vi "LoadAndAlignMulti.vi"(8 "error in (no error)":errorcluster, 11 "FileList":string[][](array[string])) -> (0 "error out":errorcluster, 3 "AllDataArray":T1[](array[typedef]) {"FlukeData"."DataAnalysisArray"."TimeStamp" format="%^<%.3X\n%x>T"; "FlukeData"."ModelDataArray"."FREQUENCY" format="%#_6f"; "FlukeData"."ModelDataArray"."TimeStamp" format="%^<%.3X\n%x>T"; "FlukeData"."PMUDataArray"."FREQUENCY" format="%#_6f"; "FlukeData"."PMUDataArray"."TimeStamp" format="%^<%.3X\n%x>T"; "NISTData"."DataAnlysisArray"."Time" format="%.6f"; "NISTData"."DataAnlysisArray"."TimeStamp" format="%^<%.3X\n%x>T"; "NISTData"."DUTDataArray"."TimeStamp" format="%^<%.3X\n%x>T"; "NISTData"."DUTDataArray"."Time" format="%.6f"; "NISTData"."NIDataArray"."TimeStamp" format="%^<%.3X\n%x>T"; "NISTData"."NIDataArray"."Time" format="%.6f"})   [LabVIEW 2014]
uses:
  typedefs/NIData.ctl
  typedefs/NIDataArray.ctl
  typedefs/PhasorRectangular.ctl
  typedefs/PmuRawDataCluster.ctl
  typedefs/CalcPhasorError.ctl
  typedefs/CalcAnalysis.ctl
  typedefs/PlotDataArrays.ctl
  typedefs/DUTData.ctl
  typedefs/NISTData.ctl
  typedefs/Alldata.ctl
  typedefs/NICalcAnalysis.ctl
  Fluke(lib)/Fluke(lib).lvlib
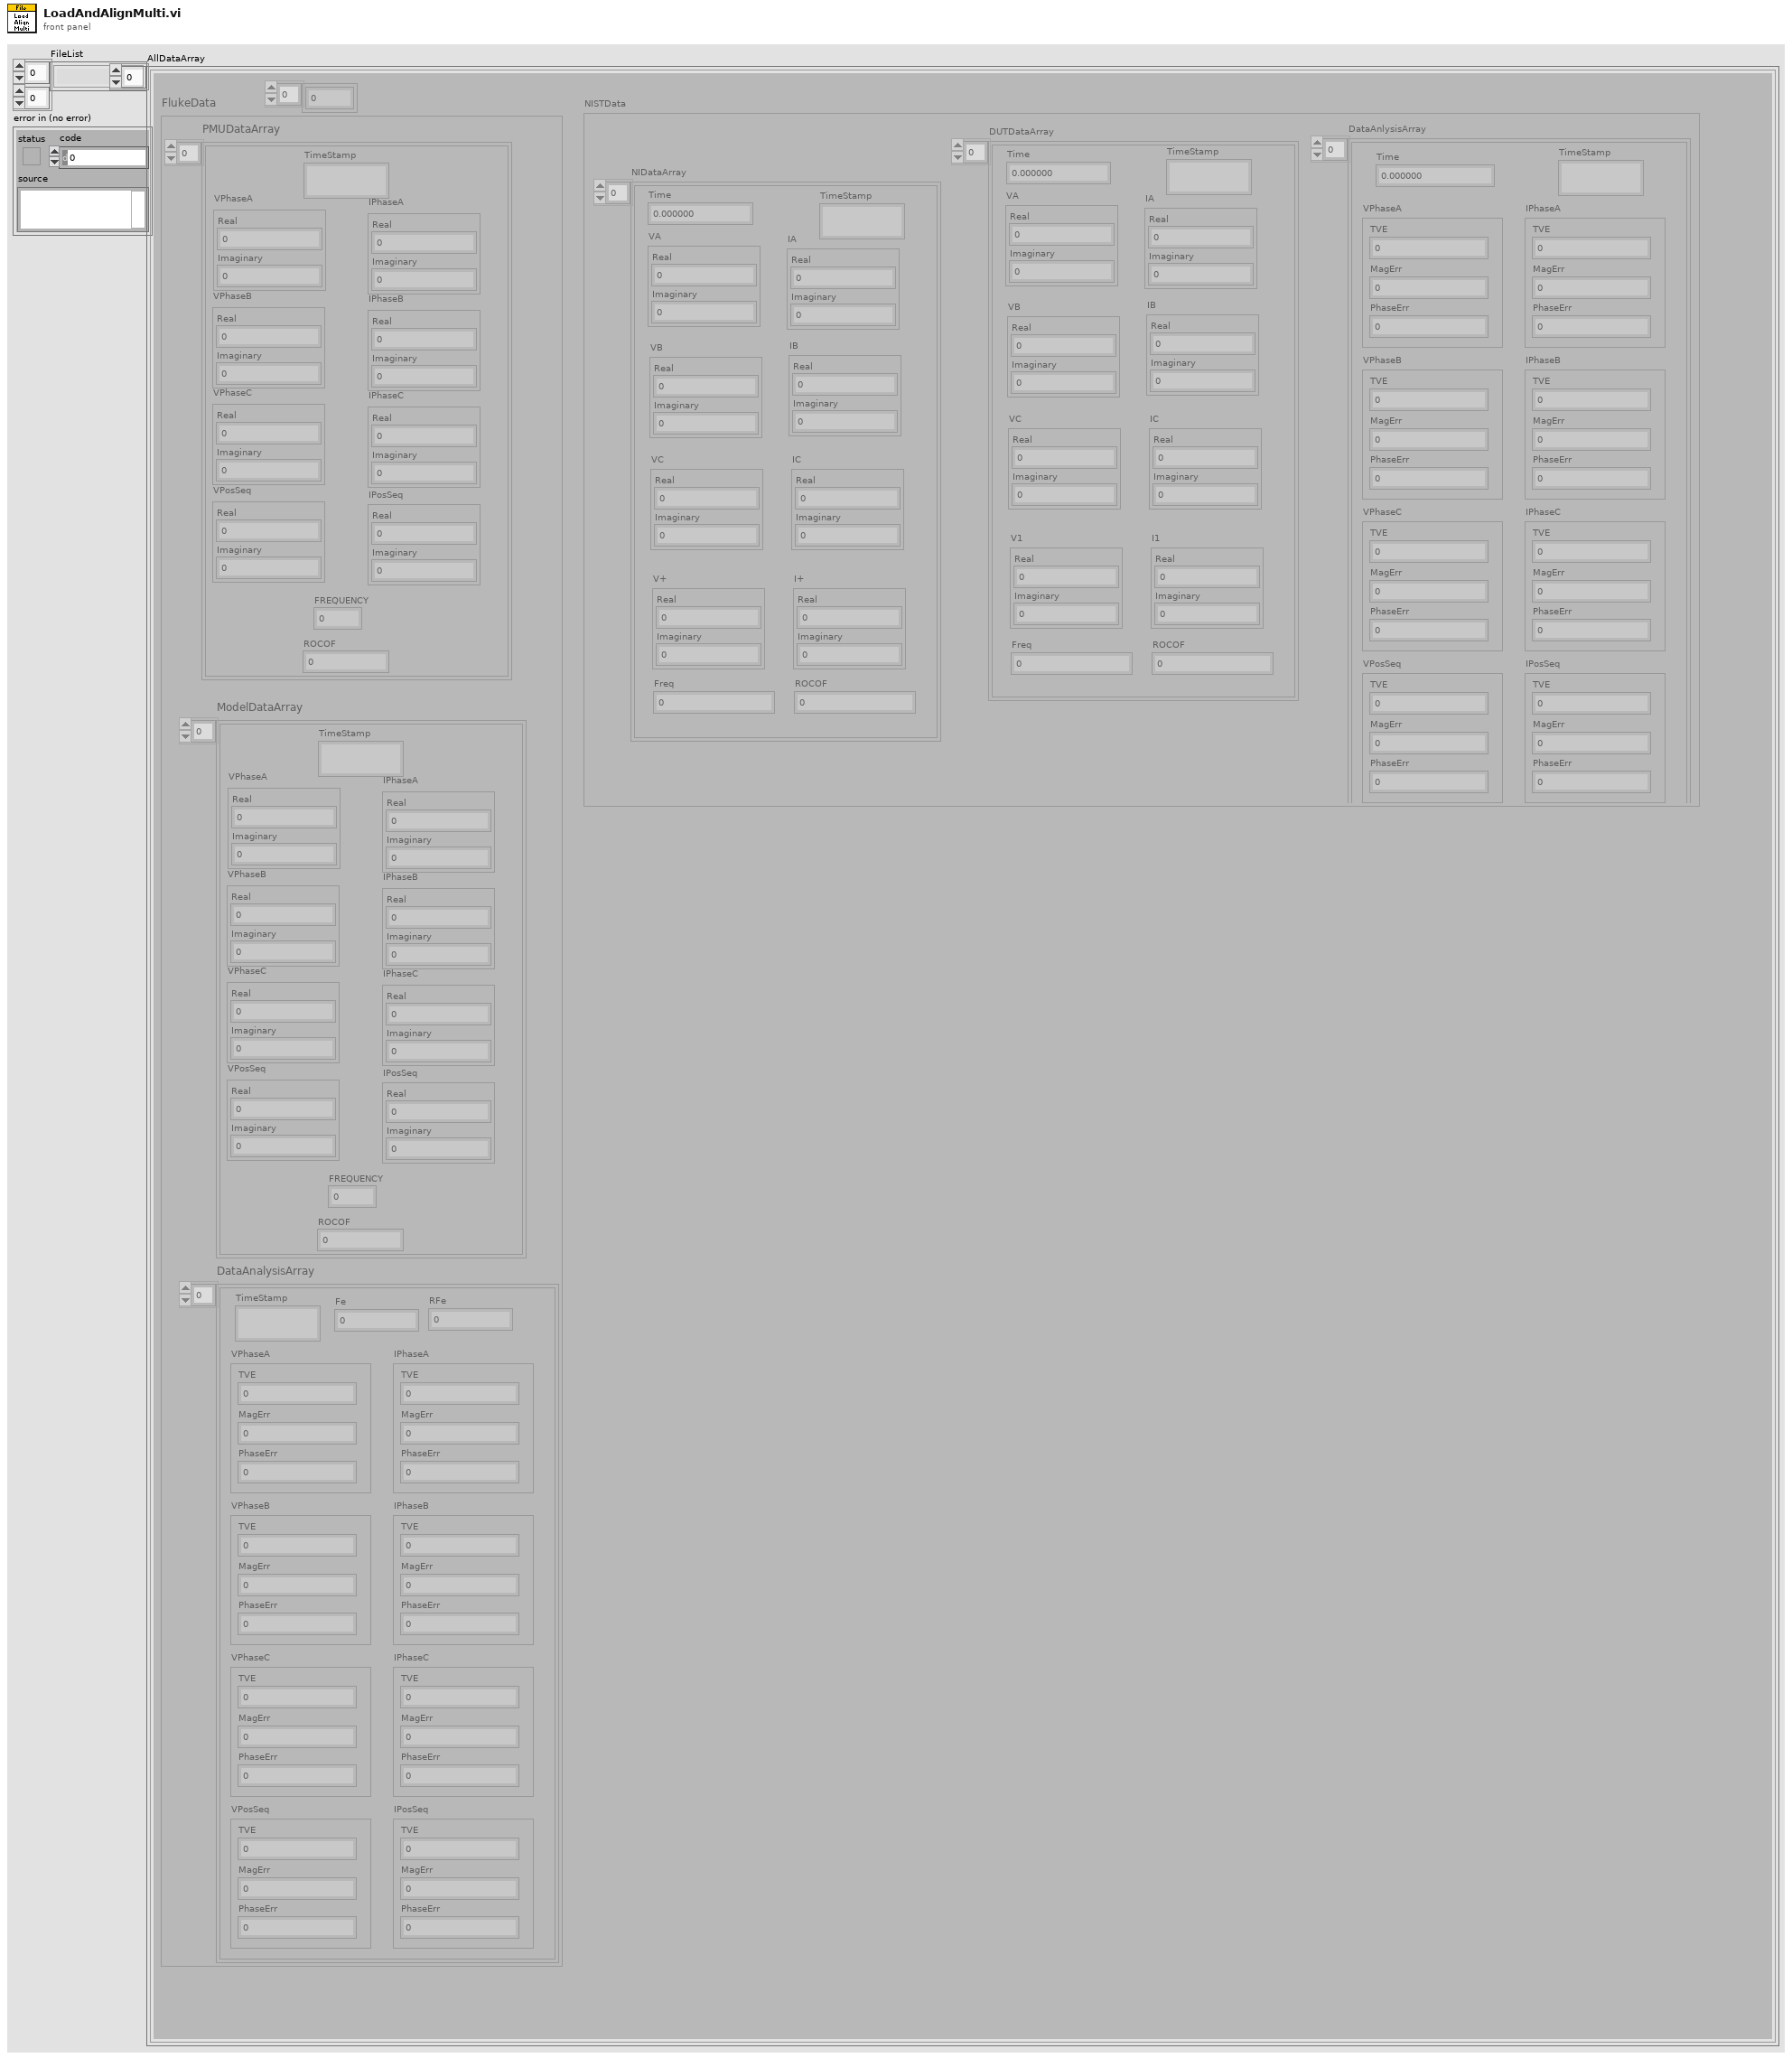
[diagram p1: front panel]
types:
  T1 = typedef "Alldata.ctl" = cluster{"NISTData":T2, "FlukeData":T9, "Params":dbl[]}
  T2 = typedef "NISTData.ctl" = cluster{"NIDataArray":T3, "DUTDataArray":T6[], "DataAnlysisArray":T7[]}
  T3 = typedef "NIDataArray.ctl" = T4[]
  T4 = typedef "NIData.ctl" = cluster{"Time":dbl, "VA":T5, "VB":T5, "VC":T5, "V+":T5, "IA":T5, "IB":T5, "IC":T5, "I+":T5, "Freq":dbl, "ROCOF":dbl, "TimeStamp":timestamp}
  T5 = typedef "PhasorRectangular.ctl" = cluster{"Real":dbl, "Imaginary":dbl}
  T6 = typedef "DUTData.ctl" = cluster{"Time":dbl, "VA":T5, "VB":T5, "VC":T5, "V1":T5, "IA":T5, "IB":T5, "IC":T5, "I1":T5, "Freq":dbl, "ROCOF":dbl, "TimeStamp":timestamp}
  T7 = typedef "NICalcAnalysis.ctl" = cluster{"Time":dbl, "VPhaseA":T8, "VPhaseB":T8, "VPhaseC":T8, "VPosSeq":T8, "IPhaseA":T8, "IPhaseB":T8, "IPhaseC":T8, "IPosSeq":T8, "Fe":dbl, "RFe":dbl, "TimeStamp":timestamp}
  T8 = typedef "CalcPhasorError.ctl" = cluster{"TVE":dbl, "MagErr":dbl, "PhaseErr":dbl}
  T9 = typedef "PlotDataArrays.ctl" = cluster{"PMUDataArray":T10[], "ModelDataArray":T10[], "DataAnalysisArray":T11[]}
  T10 = typedef "PmuRawDataCluster.ctl" = cluster{"TimeStamp":timestamp, "VPhaseA":T5, "VPhaseB":T5, "VPhaseC":T5, "VPosSeq":T5, "IPhaseA":T5, "IPhaseB":T5, "IPhaseC":T5, "IPosSeq":T5, "FREQUENCY":dbl, "ROCOF":sgl}
  T11 = typedef "CalcAnalysis.ctl" = cluster{"TimeStamp":timestamp, "VPhaseA":T8, "VPhaseB":T8, "VPhaseC":T8, "VPosSeq":T8, "IPhaseA":T8, "IPhaseB":T8, "IPhaseC":T8, "IPosSeq":T8, "Fe":dbl, "RFe":dbl}
  T12 = typedef "Fluke(lib).lvlib/TestParams.ctl" = cluster{"TestType":dbl, "F0":dbl, "Fs":dbl, "Fin":dbl, "dF":dbl, "Pin":dbl, "Iin":dbl, "Ki":dbl, "Vin":dbl, "Kv":dbl, "Fh":dbl, "Kh":dbl, "Ph":dbl, "Fi":dbl, "Kintr":dbl, "Pi":dbl, "Fx":dbl, "Kx":dbl, "Px":dbl, "Fa":dbl, "Ka":dbl, "Pa":dbl, "Sec":dbl, "Reports":dbl, "Frac":dbl, "Divisor":dbl}
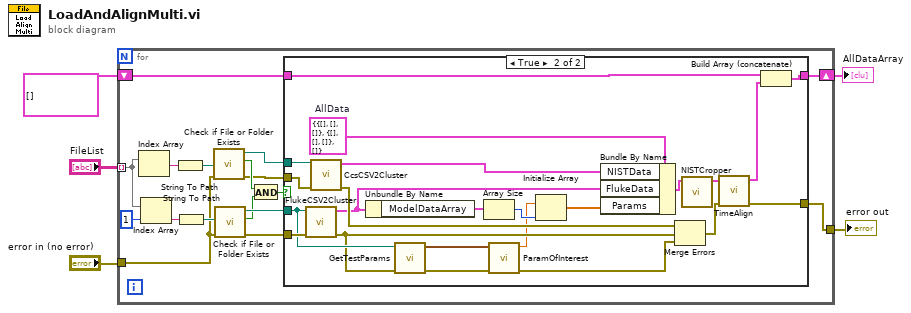
[diagram p0: block diagram]
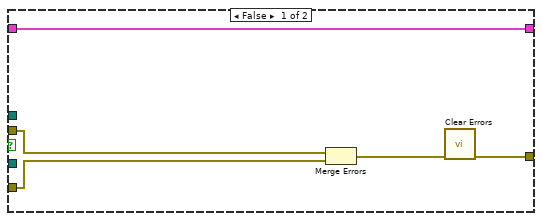
[diagram p2: hidden frame]
diagram:
  n1 = for {
    tunnel: "FileList" -> [w22] mode=indexing
    tunnel: "error in (no error)" -> [w8]
    tunnel: [w16] -> w3
    shift-right: [w9] -> w1
    shift-left: T1[] [] -> [w10]
    n2 = Index Array(array=w22) -> (element=w19:string)  [unwired: 1 in]
    n3 = Index Array(array=w22, index=1) -> (element=w20:string)
    n4 = String To Path(string=w19) -> (path=w18:path)
    n5 = String To Path(string=w20) -> (path=w17:path)
    n6 = call <vilib>:"Check if File or Folder Exists.vi"("error in (no error)"=w8, "path"=w18) -> ("error out"=w7:errorcluster, "file or folder exists?"=w12:bool, "dup path"=w15:path)  [unwired: 7 in]
    n7 = call <vilib>:"Check if File or Folder Exists.vi"("error in (no error)"=w8, "path"=w17) -> ("error out"=w6:errorcluster, "file or folder exists?"=w13:bool, "dup path"=w14:path)  [unwired: 7 in]
    n8 = And(x=w12, y=w13) -> (x .and. y?=w11:bool)
    n9 = case shown="True" w11 {
      tunnel: [w23 w46] -> w16
      tunnel: w15 -> [_ w45]
      tunnel: w14 -> [_ w37]
      tunnel: w10 -> [w27 w43]
      tunnel: [w27 w42] -> w9
      tunnel: w7 -> [w26 w41]
      tunnel: w6 -> [w25 w40]
      frame False {
        n10 = Merge Errors(w26, w25) -> (w24:errorcluster)
        n11 = call <vilib>:"Clear Errors.vi"("error in (no error)"=w24) -> ("error out"=w23:errorcluster)  [unwired: 5 in, 1 out]
      }
      frame True {
        w49 = T1 {"NISTData"={"NIDataArray"=[], "DUTDataArray"=[], "DataAnlysisArray"=[]}, "FlukeData"={"PMUDataArray"=[], "ModelDataArray"=[], "DataAnalysisArray"=[]}, "Params"=[]}  # AllData
        n12 = call "FlukeCSV2Cluster.vi"("error in (no error)"=w40, "FlukePath"=w37) -> ("error out"=w34:errorcluster, "AllDataArrays"=w32:T9)  [unwired: 8 in]
        n13 = call "CcsCSV2Cluster.vi"("error in (no error)"=w41, "CCSPath"=w45) -> ("error out"=w50:errorcluster, "AllDataArrays"=w48:T2)  [unwired: 8 in]
        n14 = Unbundle By Name(w32) -> ("ModelDataArray"=w31:T10[])
        n15 = call "GetTestParams.vi"("error in (no error)"=w34, "RawData Filename"=w37) -> ("error out"=w35:errorcluster, "TestParams"=w36:T12)  [unwired: 8 in]
        n16 = Array Size(array=w31) -> (size(s)=w29:i32)
        n17 = call "ParamOfInterest.vi"("error in (no error)"=w35, "TestParams"=w36) -> ("error out"=w33:errorcluster, "Param"=w28:dbl)  [unwired: 8 in]
        n18 = Initialize Array(w28, w29) -> (w30:dbl[])
        n19 = Bundle By Name(cluster=w49, "NISTData"=w48, "FlukeData"=w32, "Params"=w30) -> (w39:T1)
        n20 = Merge Errors(w50, w34, w33) -> (w47:errorcluster)
        n21 = call "NISTCropper.vi"("AllData In"=w39) -> ("AllData Out"=w38:T1)  [unwired: 10 in]
        n22 = call "TimeAlign.vi"("error in (no error)"=w47, "AllData In"=w38) -> ("error out"=w46:errorcluster, "AllData Out"=w44:T1)  [unwired: 8 in]
        n23 = Build Array (concatenate)(w43, w44) -> (w42:T1[])
      }
    }
  }
  "error out" <- w3
  "AllDataArray" <- w1
